vi "Main IU.vi"() -> ()   [LabVIEW 2017]
uses:
  <vilib>/Analysis/NI_AALBase.lvlib
  <vilib>/Analysis/baseanly.llb/Mean (DBL).vi
panel:
  out "SetpointVsSalida 2":cluster{"Double":dbl, "Output":dbl}(graph)
  in  "Setpoint1":dbl=1.0 min=-6.2 max=6.2 step=0.2
  in  "tetha_f_p":dbl
  in  "tetha_o_p":dbl
  in  "tetha_o_pp":dbl
  in  "tetha_f_pp":dbl
  in  "tf":dbl
  in  "Homing":bool
  out "EsfuerzoSat":dbl(graph)
  out "EsfuerzoSat2":dbl(graph)
  in  "Setpoint 2":dbl min=-1.0 max=1.0 step=0.01
  out "SetpointVsSalida":cluster{"Double":dbl, "Output":dbl}(graph)
  out "Saving Data":bool
  in  "Record Button":bool
  in  "Filename":path=path "test.lvm"
  out "Motor1":waveform(dbl)[](graph)
  in  "Paro Emergencia:\nUI y RT":bool
  in  "Stop UI":bool
  # "rad"
  # "rad/s"
  # "rad/s^2"
  # "rad/s"
  # "rad/s^2"
  # "s"
  # "rad"
  # "rad"
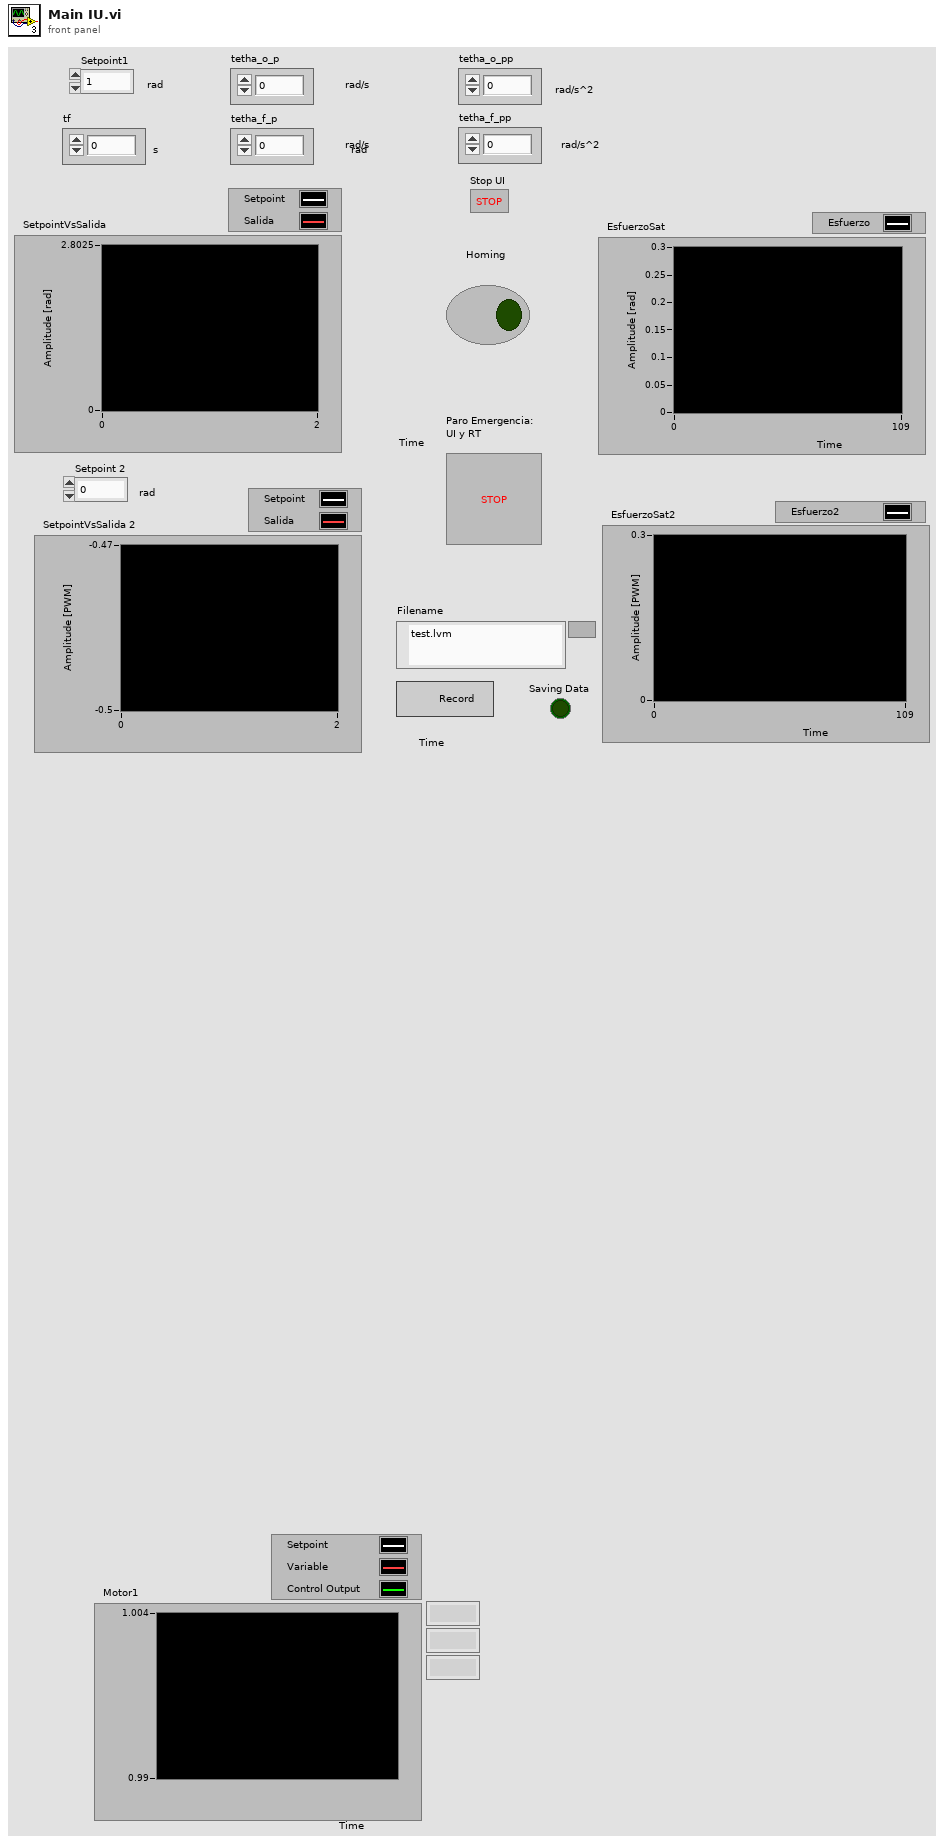
[diagram p1: front panel]
types:
  T1 = cluster{"Double":dbl, "dbl Scaled Value":dbl, "Output":dbl, "seconds since 1Jan1904":timestamp, dbl, dbl, dbl}
  T2 = cluster{"[0]":dbl, "[1]":dbl, "[2]":dbl, "[3]":dbl, "[4]":dbl, "[5]":dbl, "[6]":dbl, "[7]":dbl, "[8]":dbl}
  T3 = cluster{"writer name":string, "Variant":variant, "Variant":variant}
  T4 = cluster{"Double":dbl, "dbl Scaled Value":dbl, "Output":dbl, "seconds since 1Jan1904":timestamp, dbl, dbl, dbl}[]
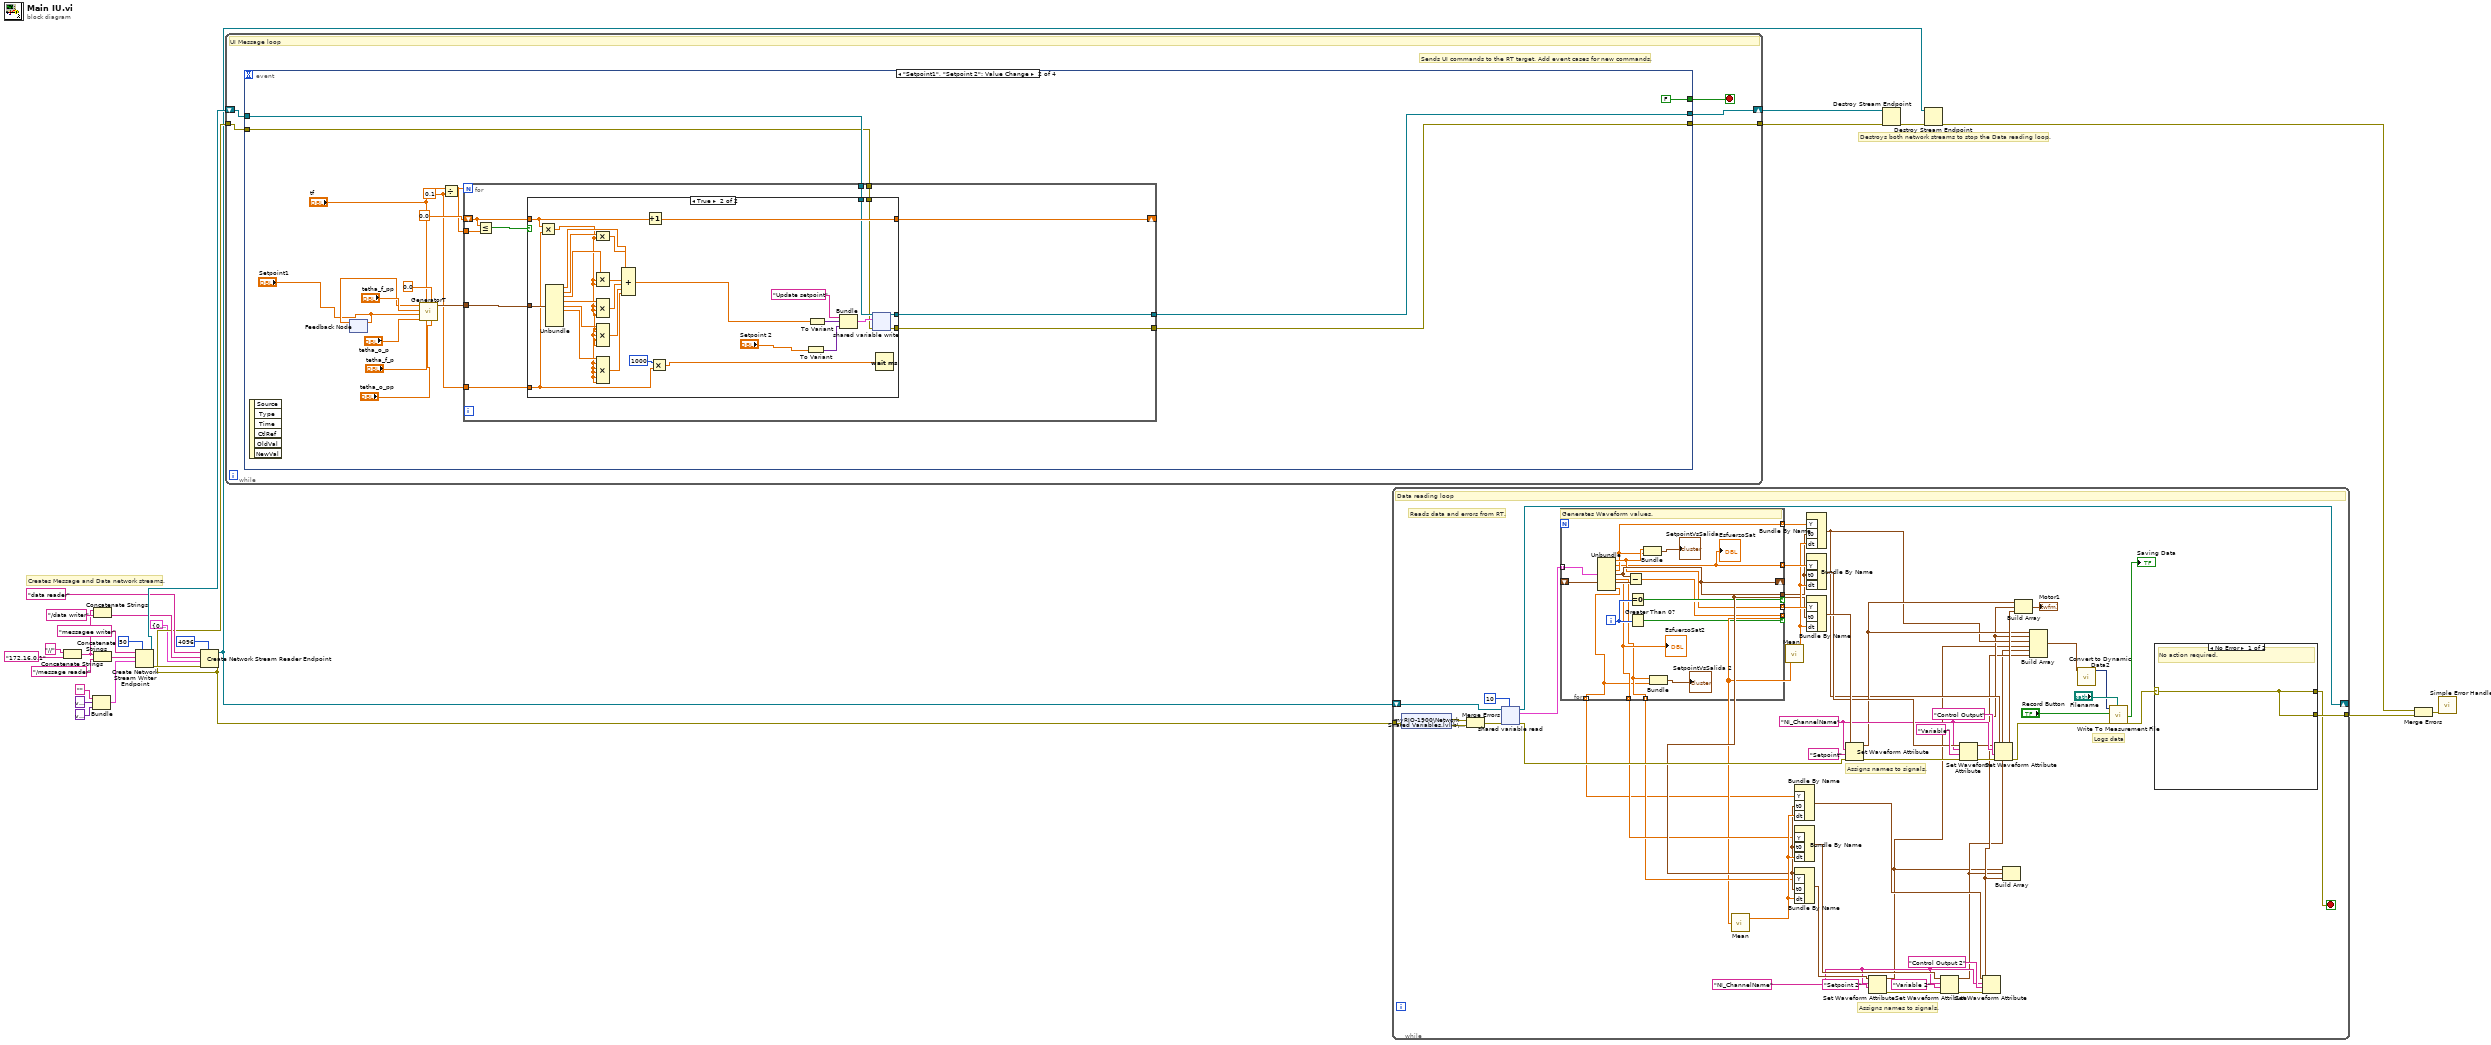
[diagram p0: block diagram]
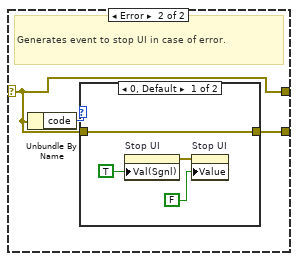
[diagram p2: hidden frame]
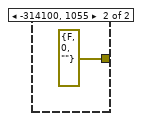
[diagram p3: hidden frame]
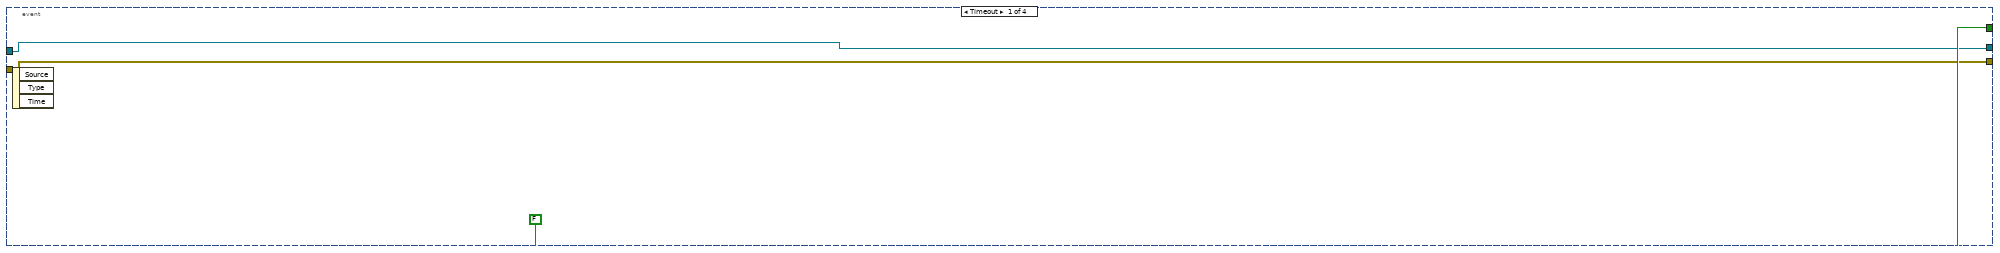
[diagram p4: hidden frame]
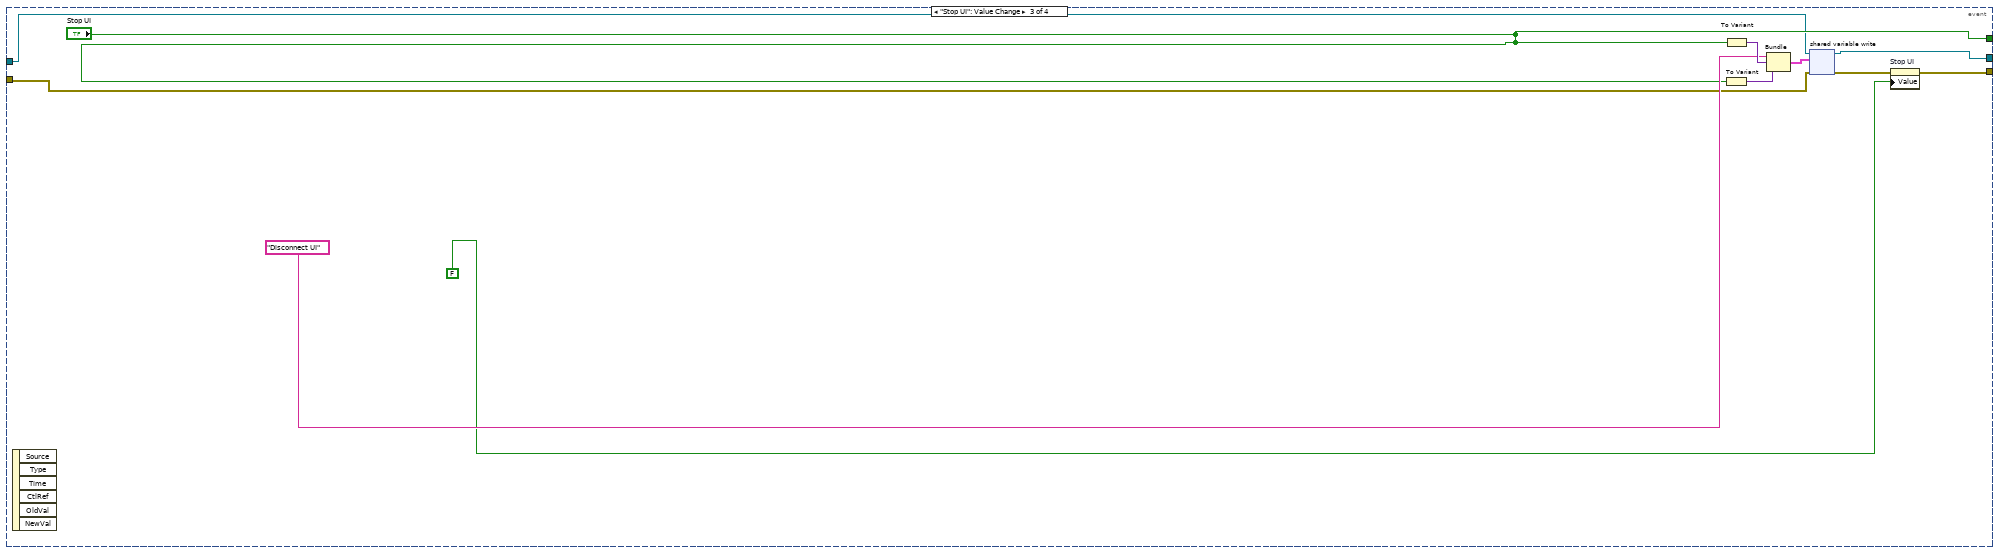
[diagram p6: hidden frame]
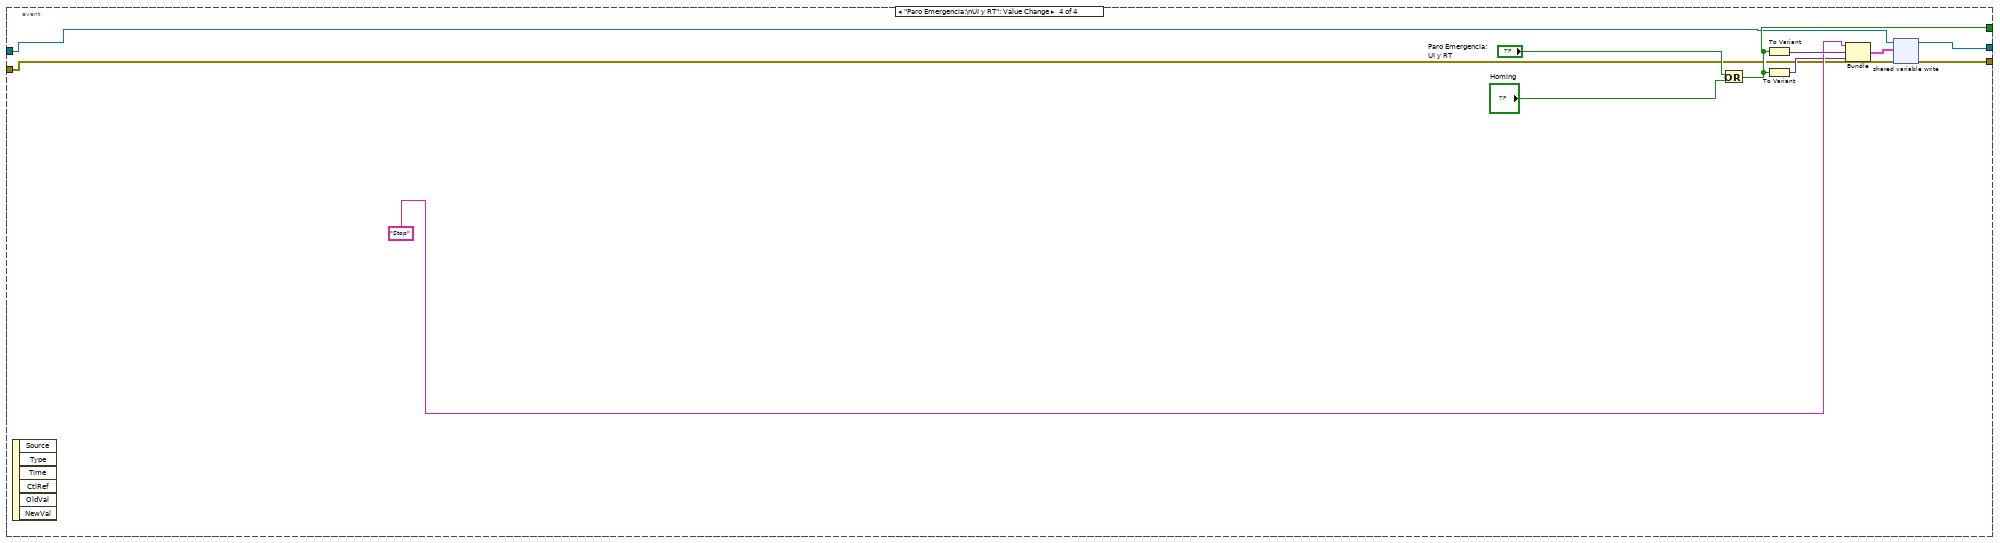
[diagram p7: hidden frame]
diagram:
  # "Destroys both network streams to stop the Data reading loop."
  # "Creates Message and Data network streams."
  n1 = Concatenate Strings("//", "172.16.0.1" ("myRIO IP")) -> (w2:string)
  n2 = Bundle("", variant, variant) -> (w26:cluster{string, variant, variant})  [unwired: 1 in]
  n3 = Concatenate Strings(w2, "/data writer") -> (w17:string)
  n4 = Concatenate Strings(w2, "/message reader") -> (w3:string)
  n5 = Create Network Stream Writer Endpoint(7:50 ("writer buffer size"), 9:w26, 10:w3, 11:"messagee writer" ("writer name")) -> (0:w14:errorcluster, 3:w20:refnum<k21>)  [unwired: 3 in]
  n6 = Create Network Stream Reader Endpoint(7:4096 ("reader buffer size"), 8:w14, 9:T1 {"Double"=0.0, "dbl Scaled Value"=0.0, "Output"=0.0, "seconds since 1Jan1904"=timestamp(0 s since 1904-01-01), 0.0, 0.0, 0.0} ("Data"), 10:w17, 11:"data reader" ("reader name")) -> (0:w13:errorcluster, 3:w6:refnum<k21>)  [unwired: 2 in]
  n7 = while {
    tunnel: w13 -> [w27]
    shift-right: [w31] -> w8
    shift-left: w20 -> [w28]
    tunnel: [w30] -> w9
    stop <- w29 stop-if-true
    # "Sends UI commands to the RT target. Add event cases for new commands."
    # "UI Message loop"
    n8 = event shown="[1] \"Setpoint1\", \"Setpoint 2\": Value Change" {
      selector: _ -> [_ _ _ _]
      dyn-events: _ -> [_ _ _ _]
      timeout: _ -> [_ _ _ _]
      tunnel: [w33 w37 w100 w110] -> w31
      tunnel: [w32 w36 w97 w111] -> w30
      tunnel: [FALSE ("Stop UI and RT") FALSE ("Stop UI and RT") "Stop UI" w106] -> w29
      tunnel: w28 -> [w33 w39 w93 w105]
      tunnel: w27 -> [w32 w38 w94 w104]
      event Timeout {
        n9 = event-data() -> ()  [unwired: 1 in, 3 out]
      }
      event "Setpoint1", "Setpoint 2": Value Change {
        w41 = 0.1 ("y")
        n10 = event-data() -> ()  [unwired: 1 in, 6 out]
        n11 = feedback #1() -> (w43:dbl)  [unwired: 1 in]
        n12 = feedback-in #1("Setpoint1") -> ()
        n13 = call "GeneratorT.vi"("tetha_o_pp"="tetha_o_pp", 5:"a0"=0.0, "tetha_f_p"="tetha_f_p", 7:"a0"="tf", "tetha_o_p"="tetha_o_p", 9:"a0"="Setpoint1", "tetha_f_pp"="tetha_f_pp", 11:"a0"=w43) -> ("Cluster"=w44:T2)  [unwired: 3 in]
        n14 = Divide(x="tf", y=w41) -> (x/y=w40:dbl)
        n15 = for {
          N: w40 -> [_]
          tunnel: w44 -> [w59]
          tunnel: w40 -> [w58]
          shift-right: [w57] -> _
          shift-left: 0.0 ("y") -> [w60]
          tunnel: w41 -> [w56]
          tunnel: w39 -> [w55]
          tunnel: w38 -> [w54]
          tunnel: [w53] -> w37
          tunnel: [w52] -> w36
          n16 = Less Or Equal?(x=w60, y=w58) -> (x <= y?=w61:bool)
          n17 = case shown="True" w61 {
            tunnel: w60 -> [w64 w77]
            tunnel: w59 -> [_ w81]
            tunnel: [w64 w80] -> w57
            tunnel: w56 -> [_ w76]
            tunnel: w55 -> [w63 w70]
            tunnel: w54 -> [w62 w69]
            tunnel: [w63 w68] -> w53
            tunnel: [w62 w67] -> w52
            frame False {
            }
            frame True {
              n18 = Multiply(x=w77, y=w76) -> (x*y=w75:dbl)
              n19 = Unbundle(w81) -> ("[0]"=w82:dbl, "[1]"=w83:dbl, "[2]"=w84:dbl, "[3]"=w85:dbl, "[4]"=w86:dbl, "[5]"=w87:dbl)  [unwired: 3 out]
              n20 = Compound Arithmetic op=MULTIPLY(w83, w75) -> (w89:dbl)
              n21 = Compound Arithmetic op=MULTIPLY(w84, w75, w75) -> (w88:dbl)
              n22 = Compound Arithmetic op=MULTIPLY(w85, w75, w75, w75) -> (w90:dbl)
              n23 = Compound Arithmetic op=MULTIPLY(w86, w75, w75, w75, w75) -> (w91:dbl)
              n24 = Compound Arithmetic op=MULTIPLY(w87, w75, w75, w75, w75, w75) -> (w92:dbl)
              n25 = Compound Arithmetic op=ADD(w82, w89, w88, w90, w91, w92) -> (w66:dbl)
              n26 = Increment(x=w77) -> (x+1=w80:dbl)
              n27 = Multiply(x=u32 1000 ("milliseconds to wait"), y=w76) -> (x*y=w78:dbl)
              n28 = To Variant(anything="Setpoint 2") -> (Variant=w74:variant)
              n29 = To Variant(anything=w66) -> (Variant=w72:variant)
              n30 = Bundle("writer name"="Update setpoint", "Variant"=w72, "Variant"=w74) -> (w73:T3)  [unwired: 1 in]
              n31 = shared-variable-write(w70, w69, w73) -> (w68:refnum<k21>, w67:errorcluster)  [unwired: 1 in, 1 out]
              n32 = Wait (ms)(milliseconds to wait=w78) -> ()  [unwired: 1 out]
            }
          }
        }
      }
      event "Stop UI": Value Change {
        n33 = event-data() -> ()  [unwired: 1 in, 6 out]
        n34 = To Variant(anything="Stop UI") -> (Variant=w96:variant)
        n35 = To Variant(anything="Stop UI") -> (Variant=w103:variant)
        n36 = Bundle("writer name"="Disconnect UI", "Variant"=w103, "Variant"=w96) -> (w102:T3)  [unwired: 1 in]
        n37 = shared-variable-write(w93, w94, w102) -> (w100:refnum<k21>, w98:errorcluster)  [unwired: 1 in, 1 out]
        n38 = property on="Stop UI" class="Bool (strict)"(error in=w98, "Value"=FALSE ("Stop UI and RT")) -> (error out=w97:errorcluster)  [unwired: 1 in, 1 out]
      }
      event "Paro Emergencia:\nUI y RT": Value Change {
        n39 = event-data() -> ()  [unwired: 1 in, 6 out]
        n40 = Or(x="Paro Emergencia:\nUI y RT", y="Homing") -> (x .or. y?=w106:bool)
        n41 = To Variant(anything=w106) -> (Variant=w114:variant)
        n42 = To Variant(anything=w106) -> (Variant=w109:variant)
        n43 = Bundle("writer name"="Stop", "Variant"=w114, "Variant"=w109) -> (w113:T3)  [unwired: 1 in]
        n44 = shared-variable-write(w105, w104, w113) -> (w110:refnum<k21>, w111:errorcluster)  [unwired: 1 in, 1 out]
      }
    }
  }
  n45 = while {
    tunnel: w13 -> [w142]
    shift-right: [w152] -> _
    shift-left: w6 -> [w167]
    tunnel: [w141] -> w10
    stop <- w140 stop-if-true
    w129 = "NI_ChannelName" ("name")
    w146 = "NI_ChannelName" ("name")
    # "Assigns names to signals."
    # "Logs data"
    # "Assigns names to signals."
    # "Reads data and errors from RT."
    # "Data reading loop"
    n46 = shared-variable "myRIO-1900\\Network Shared Variables.lvlib\\error IO"(error in=w142) -> (w145:errorcluster, error out=w144:errorcluster)
    n47 = Merge Errors(w145, w144) -> (w143:errorcluster)
    n48 = shared-variable-read(w167, w143, 10 ("# elements")) -> (w152:refnum<k21>, w157:errorcluster, w165:T4)  [unwired: 1 in, 1 out]
    n49 = for {
      tunnel: w165 -> [w191] mode=indexing
      tunnel: [w184] -> w164 mode=indexing
      tunnel: [w181] -> w163 mode=indexing
      tunnel: [w183] -> w139 mode=indexing
      tunnel: [w189] -> w128 if=w190
      shift-right: [w189] -> _
      shift-left: _ -> [w188]
      tunnel: [w187] -> w125 mode=indexing if=w185
      tunnel: [w177] -> w124 mode=indexing
      tunnel: [w180] -> w127 mode=indexing
      tunnel: [w178] -> w126 mode=indexing
      i -> [w186]
      # "Generates Waveform values."
      n50 = Unbundle(w191) -> ("Double"=w184:dbl, "dbl Scaled Value"=w181:dbl, "Output"=w183:dbl, "seconds since 1Jan1904"=w189:timestamp, w178:dbl, w180:dbl, w177:dbl)
      "EsfuerzoSat2" <- w180
      "EsfuerzoSat" <- w181
      n51 = Subtract(x=w189, y=w188) -> (x-y=w187:dbl)
      n52 = Equal To 0?(x=w186) -> (x = 0?=w190:bool)
      n53 = Greater Than 0?(x=w186) -> (x > 0?=w185:bool)
      n54 = Bundle("Double"=w184, "Output"=w183) -> (→"SetpointVsSalida":cluster{"Double":dbl, "Output":dbl})  [unwired: 1 in]
      n55 = Bundle(w178, w177) -> (→"SetpointVsSalida 2":cluster{dbl, dbl})  [unwired: 1 in]
    }
    n56 = call-poly <vilib>:"Mean.vi"("X"=w125) -> ("mean"=w138:dbl)  [unwired: 1 out]
    n57 = call-poly <vilib>:"Mean.vi"("X"=w125) -> ("mean"=w162:dbl)  [unwired: 1 out]
    n58 = Bundle By Name("Y"=w124, "t0"=w128, "dt"=w138) -> (w130:waveform(dbl))  [unwired: 1 in]
    n59 = Bundle By Name("Y"=w127, "t0"=w128, "dt"=w138) -> (w131:waveform(dbl))  [unwired: 1 in]
    n60 = Bundle By Name("Y"=w126, "t0"=w128, "dt"=w138) -> (w137:waveform(dbl))  [unwired: 1 in]
    n61 = Bundle By Name("Y"=w139, "t0"=w128, "dt"=w162) -> (w120:waveform(dbl))  [unwired: 1 in]
    n62 = Bundle By Name("Y"=w163, "t0"=w128, "dt"=w162) -> (w154:waveform(dbl))  [unwired: 1 in]
    n63 = Bundle By Name("Y"=w164, "t0"=w128, "dt"=w162) -> (w161:waveform(dbl))  [unwired: 1 in]
    n64 = Set Waveform Attribute(4:w157, 5:"Setpoint" ("name"), 6:w146, 7:w161) -> (0:w156:errorcluster, 3:w121:waveform(dbl))  [unwired: 1 out]
    n65 = Set Waveform Attribute(5:"Setpoint 2" ("name"), 6:w129, 7:w137) -> (0:w133:errorcluster, 3:w116:waveform(dbl))  [unwired: 1 in, 1 out]
    n66 = Set Waveform Attribute(4:w133, 5:"Variable 2" ("name"), 6:w129, 7:w131) -> (0:w132:errorcluster, 3:w117:waveform(dbl))  [unwired: 1 out]
    n67 = Set Waveform Attribute(4:w156, 5:"Variable" ("name"), 6:w146, 7:w154) -> (0:w155:errorcluster, 3:w119:waveform(dbl))  [unwired: 1 out]
    n68 = Set Waveform Attribute(4:w132, 5:"Control Output 2" ("name"), 6:w129, 7:w130) -> (3:w118:waveform(dbl))  [unwired: 2 out]
    n69 = Set Waveform Attribute(4:w155, 5:"Control Output" ("name"), 6:w146, 7:w120) -> (0:w151:errorcluster, 3:w153:waveform(dbl))  [unwired: 1 out]
    n70 = Build Array(w116, w117, w118) -> ()  [unwired: 1 out]
    n71 = Build Array(w121, w119, w153) -> (→"Motor1":waveform(dbl)[])
    n72 = Build Array(w121, w119, w120, w116, w117, w118) -> (w115:waveform(dbl)[])
    n73 = call "Convert to Dynamic Data2"("Array of Waveforms"=w115) -> ("Dynamic Data Type"=w122:dynamicdata)  [unwired: 3 in]
    n74 = call "Write To Measurement File"("Signals"=w122, "Enable"="Record Button", "error in (no error)"=w151, "Filename"="Filename") -> ("Saving Data"=→"Saving Data":bool, "error out"=w147:errorcluster)  [unwired: 13 in, 1 out]
    n75 = case shown="No Error" w147 {
      selector: w147 -> [w168 w169]
      tunnel: [w168 w170] -> w141
      tunnel: [w168 w169] -> w140
      frame No Error {
        # "No action required."
      }
      frame Error {
        # "Generates event to stop UI in case of error."
        n76 = Unbundle By Name(w169) -> ("code"=w171:i32)
        n77 = case shown="0, Default" w171 {
          tunnel: [w174 errorcluster {"status"=FALSE, "code"=0, "source"=""} ("error IO")] -> w170
          tunnel: w169 -> [w174 _]
          frame 0, Default {
            n78 = property on="Stop UI" class="Bool (strict)"("Val(Sgnl)"=TRUE ("Stop UI and RT")) -> (error out=w173:errorcluster)  [unwired: 2 in, 1 out]
            n79 = property on="Stop UI" class="Bool (strict)"(error in=w173, "Value"=FALSE ("Stop UI")) -> ()  [unwired: 1 in, 2 out]
          }
          frame -314100, 1055 {
          }
        }
      }
    }
  }
  n80 = Destroy Stream Endpoint(8:w9, 11:w8) -> (0:w7:errorcluster)
  n81 = Destroy Stream Endpoint(8:w7, 11:w6) -> (0:w5:errorcluster)
  n82 = Merge Errors(w5, w10) -> (w11:errorcluster)
  n83 = call <vilib>:"Simple Error Handler.vi"("error in (no error)"=w11) -> ()  [unwired: 4 in, 5 out]
